vi "Get Stream Position.vi"(8 "error in (no error)":errorcluster, 11 "StringStream in":refnum<class "StringStream.lvclass">) -> (0 "error out":errorcluster, 2 "Position":i64, 3 "StringStream out":refnum<class "StringStream.lvclass">)   [LabVIEW 2020, in "Stream.lvlib" / "StringStream.lvclass"]
uses:
  StringStream.lvclass
  StringStream.lvclass/StringStream.ctl
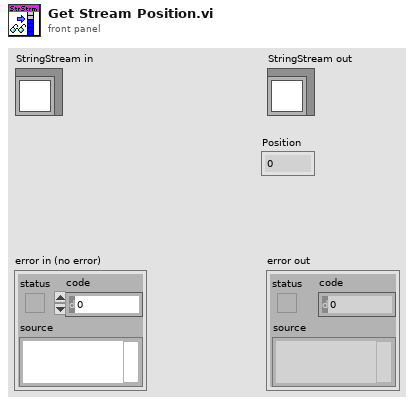
[diagram p1: front panel]
types:
  T1 = typedef "Stream.lvlib/StringStream.lvclass/Ref Data.ctl" = cluster{"Position":i64, "String":string}
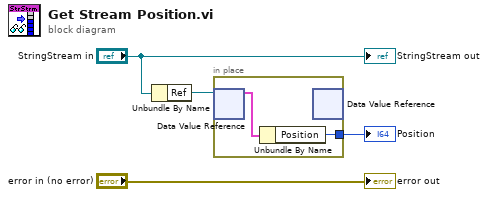
[diagram p0: block diagram]
diagram:
  n1 = Unbundle By Name("StringStream in") -> ("Ref"=w3:refnum<data-value>)
  n2 = in-place {
    in-place-border: [w5] -> w1
    n3 = in-place-dvr #1(w3) -> (w6:T1)  [unwired: 1 out]
    n4 = Unbundle By Name(w6) -> ("Position"=w5:i64)
    n5 = in-place-dvr #1() -> ()  [unwired: 1 in, 2 out]
  }
  "Position" <- w1
  "error out" <- "error in (no error)"
  "StringStream out" <- "StringStream in"
